vi "Read Eye Params.vi"(8 "error in (no error)":errorcluster, 11 "TrialBasedExperiment in":refnum<class "MatlabExperiment.lvclass">) -> (0 "error out":errorcluster, 2 "Eye Params":dbl[](array[numeric]), 3 "TrialBasedExperiment out":refnum<class "MatlabExperiment.lvclass">)   [LabVIEW 2010]
uses:
  TrialBasedExperimentObject/Eye Params.vi
  MatlabExperiment.lvclass
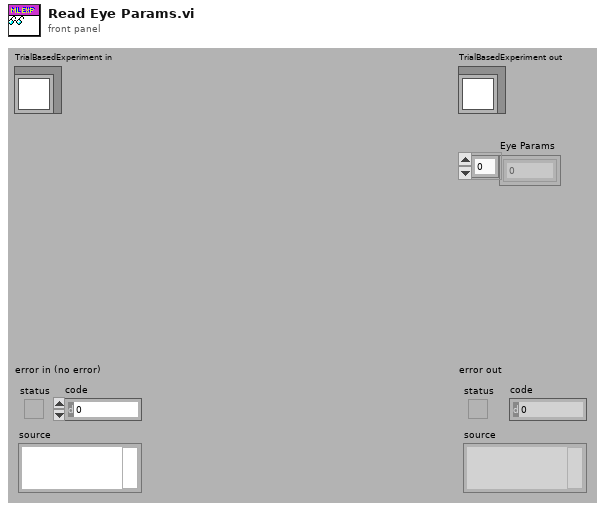
[diagram p1: front panel]
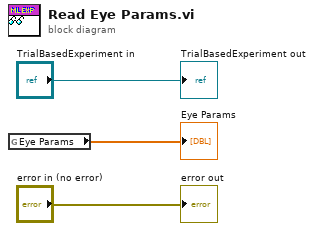
[diagram p0: block diagram]
diagram:
  n1 = global read "Eye Params.vi" "Eye Params"() -> (→"Eye Params":dbl[])
  "error out" <- "error in (no error)"
  "TrialBasedExperiment out" <- "TrialBasedExperiment in"
